vi "Place a dot on each strip and center.vi"(0 "Image":T1, 1 "Avg Factor":i32=1, 5 "x1 (L) IN":dbl, 7 "y1 (L) IN":dbl, 9 "x2 (R) IN":dbl, 11 "y2 (R) IN":dbl) -> (4 "Image Out":T1, 6 "x1 (L) out":dbl, 8 "y1 (L) out":dbl, 10 "x2 (R) out":dbl, 15 "y2 (R) out":dbl)   [LabVIEW 2018]
uses:
  <vilib>/vision/Image Controls.llb/IMAQ Image.ctl
  <vilib>/ptbypt/NI_PtbyPt.lvlib
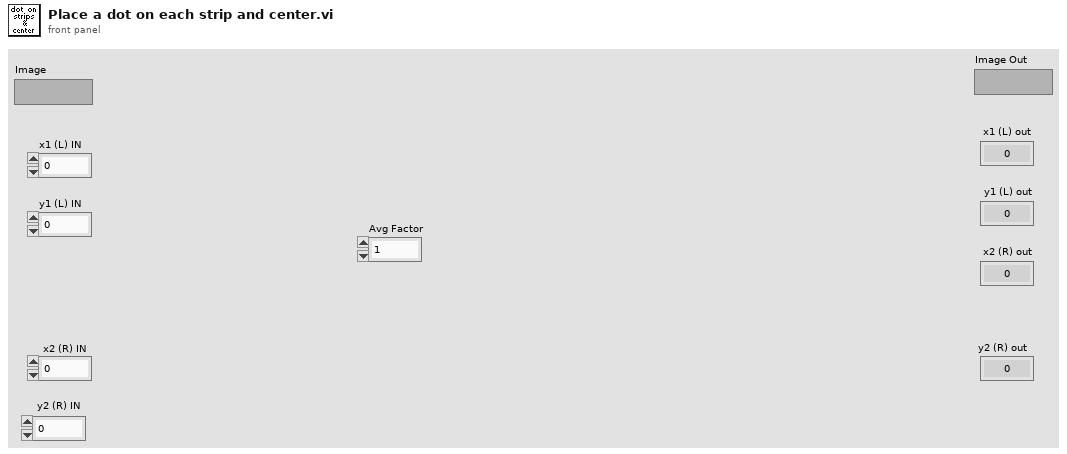
[diagram p1: front panel]
types:
  T1 = typedef "IMAQ Image.ctl" = refnum<image>
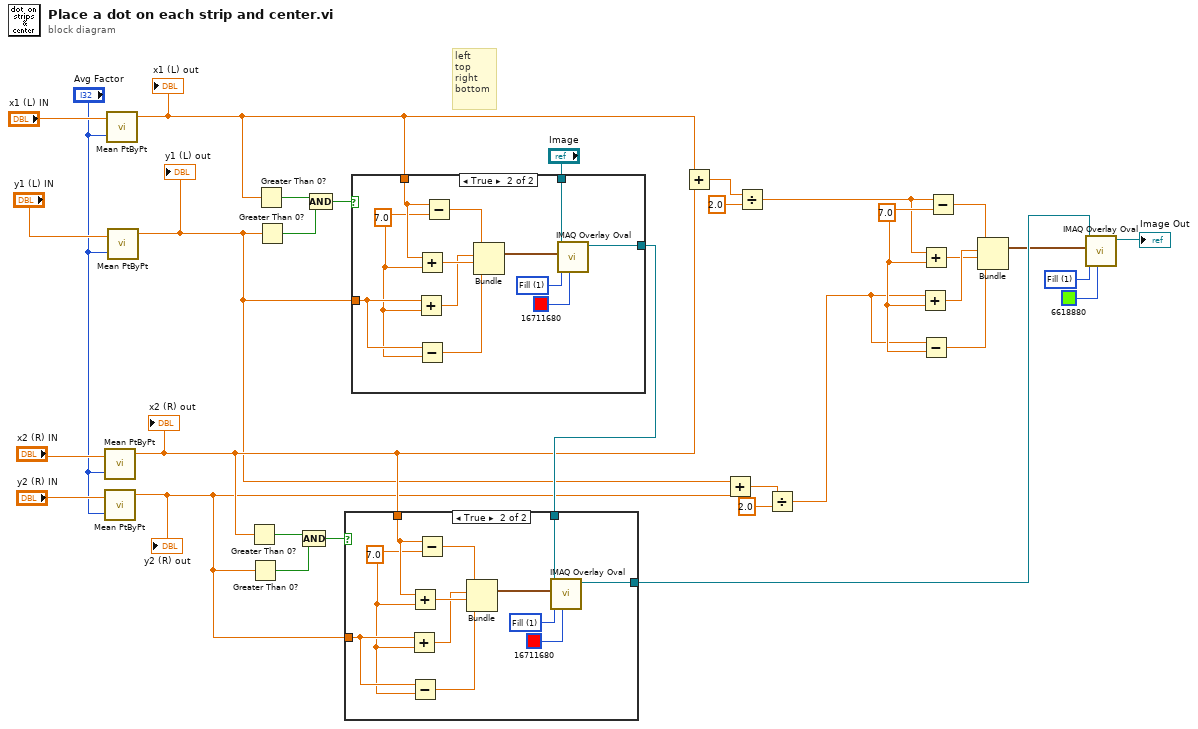
[diagram p0: block diagram]
diagram:
  w4 = u32 1 items=["Frame", "Fill"] ("Drawing Mode (Frame)")
  w17 = 7.0 ("y")
  # "left\ntop\nright\nbottom"
  n1 = call <vilib>:"Mean PtByPt.vi"("x"="x2 (R) IN", "sample length"="Avg Factor") -> ("mean"=w19:dbl)  [unwired: 2 in, 1 out]
  "x2 (R) out" <- w19
  n2 = call <vilib>:"Mean PtByPt.vi"("x"="y2 (R) IN", "sample length"="Avg Factor") -> ("mean"=w9:dbl)  [unwired: 2 in, 1 out]
  "y2 (R) out" <- w9
  n3 = call <vilib>:"Mean PtByPt.vi"("x"="x1 (L) IN", "sample length"="Avg Factor") -> ("mean"=w20:dbl)  [unwired: 2 in, 1 out]
  "x1 (L) out" <- w20
  n4 = call <vilib>:"Mean PtByPt.vi"("x"="y1 (L) IN", "sample length"="Avg Factor") -> ("mean"=w10:dbl)  [unwired: 2 in, 1 out]
  "y1 (L) out" <- w10
  n5 = Greater Than 0?(x=w19) -> (x > 0?=w22:bool)
  n6 = Greater Than 0?(x=w9) -> (x > 0?=w23:bool)
  n7 = Greater Than 0?(x=w20) -> (x > 0?=w28:bool)
  n8 = Greater Than 0?(x=w10) -> (x > 0?=w27:bool)
  n9 = Compound Arithmetic op=AND(w22, w23) -> (w24:bool)
  n10 = Compound Arithmetic op=AND(w28, w27) -> (w25:bool)
  n11 = case shown="True" w25 {
    tunnel: w20 -> [_ w40]
    tunnel: "Image" -> [w34 w43]
    tunnel: [w34 w42] -> w21
    tunnel: w10 -> [_ w37]
    frame False {
    }
    frame True {
      w45 = u32 1 items=["Frame", "Fill"] ("Drawing Mode (Frame)")
      w36 = 7.0 ("y")
      n12 = Add(x=w37, y=w36) -> (x+y=w38:dbl)
      n13 = Add(x=w40, y=w36) -> (x+y=w39:dbl)
      n14 = Subtract(x=w37, y=w36) -> (x-y=w35:dbl)
      n15 = Subtract(x=w40, y=w36) -> (x-y=w41:dbl)
      n16 = Bundle(w41, w38, w39, w35) -> (w46:cluster{dbl, dbl, dbl, dbl})  [unwired: 1 in]
      n17 = call "IMAQ Overlay Oval"("Color"=u32 16711680, "Drawing Mode (Frame)"=w45, "Bounding Rectangle"=w46, "Image"=w43) -> ("Image Out"=w42:T1)  [unwired: 6 in, 1 out]
    }
  }
  n18 = case shown="True" w24 {
    tunnel: w19 -> [_ w53]
    tunnel: w21 -> [w47 w56]
    tunnel: [w47 w55] -> w3
    tunnel: w9 -> [_ w50]
    frame False {
    }
    frame True {
      w58 = u32 1 items=["Frame", "Fill"] ("Drawing Mode (Frame)")
      w49 = 7.0 ("y")
      n19 = Add(x=w50, y=w49) -> (x+y=w51:dbl)
      n20 = Add(x=w53, y=w49) -> (x+y=w52:dbl)
      n21 = Subtract(x=w50, y=w49) -> (x-y=w48:dbl)
      n22 = Subtract(x=w53, y=w49) -> (x-y=w54:dbl)
      n23 = Bundle(w54, w51, w52, w48) -> (w59:cluster{dbl, dbl, dbl, dbl})  [unwired: 1 in]
      n24 = call "IMAQ Overlay Oval"("Color"=u32 16711680, "Drawing Mode (Frame)"=w58, "Bounding Rectangle"=w59, "Image"=w56) -> ("Image Out"=w55:T1)  [unwired: 6 in, 1 out]
    }
  }
  n25 = Add(x=w20, y=w19) -> (x+y=w13:dbl)
  n26 = Add(x=w10, y=w9) -> (x+y=w7:dbl)
  n27 = Divide(x=w13, y=2.0) -> (x/y=w11:dbl)
  n28 = Divide(x=w7, y=2.0) -> (x/y=w6:dbl)
  n29 = Add(x=w6, y=w17) -> (x+y=w16:dbl)
  n30 = Add(x=w11, y=w17) -> (x+y=w15:dbl)
  n31 = Subtract(x=w6, y=w17) -> (x-y=w18:dbl)
  n32 = Subtract(x=w11, y=w17) -> (x-y=w14:dbl)
  n33 = Bundle(w14, w16, w15, w18) -> (w2:cluster{dbl, dbl, dbl, dbl})  [unwired: 1 in]
  n34 = call "IMAQ Overlay Oval"("Color"=u32 6618880, "Drawing Mode (Frame)"=w4, "Bounding Rectangle"=w2, "Image"=w3) -> ("Image Out"=→"Image Out":T1)  [unwired: 6 in, 1 out]
